vi "GetProperties.vi"(8 "error in":errorcluster, 11 "Ring in":refnum<class "Combobox.lvclass">) -> (0 "error out":errorcluster, 3 "Ring out":refnum<class "Combobox.lvclass">)   [LabVIEW 2014, in "Raspberry Pi Compatible Compiler for LabVIEW.lvlib" / "Combobox.lvclass"]
uses:
  Combobox.lvclass
  Combobox.lvclass/Combobox.ctl
  String/String.lvclass
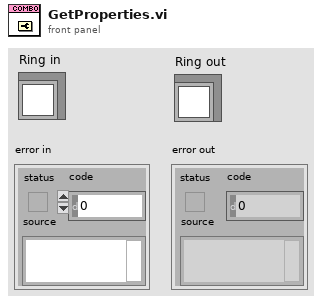
[diagram p1: front panel]
types:
  T1 = typedef "LVComboBoxStrsAndValuesArrayTypeDef.ctl" = cluster{"String":string, "Value":string}[]
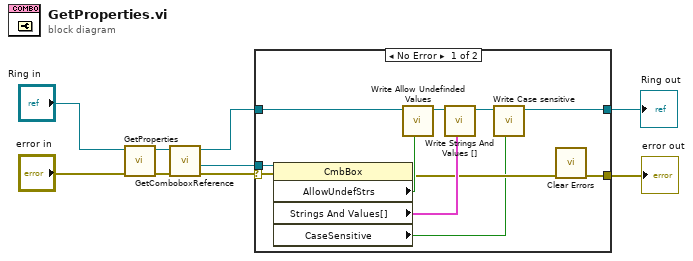
[diagram p0: block diagram]
diagram:
  n1 = call-parent "GetProperties.vi"("error in"="error in", "String in"="Ring in") -> ("error out"=w6:errorcluster, "String out"=w7:refnum<class "Combobox.lvclass">)  [unwired: 8 in]
  n2 = call "GetComboboxReference.vi"("error in"=w6, "Combobox in"=w7) -> ("error out"=w5:errorcluster, "Combobox reference"=w4:refnum<vi>, "Combobox out"=w3:refnum<class "Combobox.lvclass">)  [unwired: 7 in]
  n3 = case shown="No Error" w5 {
    selector: w5 -> [w20 w21]
    tunnel: w4 -> [w19 _]
    tunnel: w3 -> [w17 w22]
    tunnel: [w10 w21] -> w1
    tunnel: [w12 w22] -> w2
    frame No Error {
      n4 = property class="CmbBox"(reference=w19, error in=w20) -> (error out=w14:errorcluster, "AllowUndefStrs"=w18:bool, "Strings And Values[]"=w16:T1, "CaseSensitive"=w11:bool)  [unwired: 1 out]
      n5 = call "Write Allow Undefinded Values.vi"("Allow Undefinded Values"=w18, "Combobox in"=w17) -> ("Combobox out"=w15:refnum<class "Combobox.lvclass">)  [unwired: 7 in]
      n6 = call "Write Strings And Values [].vi"("Strings And Values []"=w16, "Combobox in"=w15) -> ("Combobox out"=w13:refnum<class "Combobox.lvclass">)  [unwired: 7 in]
      n7 = call "Write Case sensitive.vi"("Case sensitive"=w11, "Combobox in"=w13) -> ("Combobox out"=w12:refnum<class "Combobox.lvclass">)  [unwired: 7 in]
      n8 = call <vilib>:"Clear Errors.vi"("error in (no error)"=w14) -> ("error out"=w10:errorcluster)  [unwired: 5 in, 1 out]
    }
    frame Error {
    }
  }
  "error out" <- w1
  "Ring out" <- w2
